vi "Configure Command.vi"(8 "error in (no error)":errorcluster, 10 "settings":T2 {"Linked Channels"."Channel Ref in" format="%.0x"}, 11 "command refnum in":T1=18446744073709551615 format="%.0x") -> (0 "error out":errorcluster, 3 "command refnum out":T1=18446744073709551615 format="%.0x")   [LabVIEW 2020, in "Instrument Addon Scripting API.lvlib"]
doc: "Configures a specified command. \n\nIf you want to use Linked Channels with the Command Format string, ensure the Channel Refnums used in the Linked Channels parameter already exist before calling this SubVI. \n\nAn error will occur in the following situations:\n- The Command Format string contains duplicate Variable Names. \n- The number of variables in the Command Format string differs from the number of Linked Channels. \n- The Variable Names in the Command Format string differs from the names used in the Linked Channels parameter."
uses:
  Instrument Addon Scripting API.lvlib
  TypeDefs/Command Settings.ctl
  <vilib>/NI VeriStand/Custom Device API/Custom Device Item Ref.ctl
  TypeDefs/Padding.ctl
  Addon/Addon Shared/Types/FG Control.ctl
  Addon/Addon Shared/Types/Command Parameters.ctl
  Addon/Addon Shared/Types/Linked Channel Cluster.ctl
  Addon/Addon Shared/SubVIs/Constants.vi
  <vilib>/NI VeriStand/Custom Device API/NI VeriStand - Get Item Property.vi
  <vilib>/NI VeriStand/Custom Device API/Get Item Property (String).vi
  <vilib>/NI VeriStand/Custom Device API/Get Item Property (String Array).vi
  <vilib>/NI VeriStand/Custom Device API/Get Item Property (Boolean).vi
  <vilib>/NI VeriStand/Custom Device API/Get Item Property (U32).vi
  <vilib>/NI VeriStand/Custom Device API/NI VeriStand - Set Item Property.vi
  <vilib>/NI VeriStand/Custom Device API/Set Item Property (String).vi
  <vilib>/NI VeriStand/Custom Device API/Set Item Property (String Array).vi
  <vilib>/NI VeriStand/Custom Device API/Set Item Property (Boolean).vi
  <vilib>/NI VeriStand/Custom Device API/Set Item Property (U32).vi
  Addon/Addon Shared/Instrument Addon Shared.lvlib
  <vilib>/NI VeriStand/Custom Device API/Custom Device API.lvlib
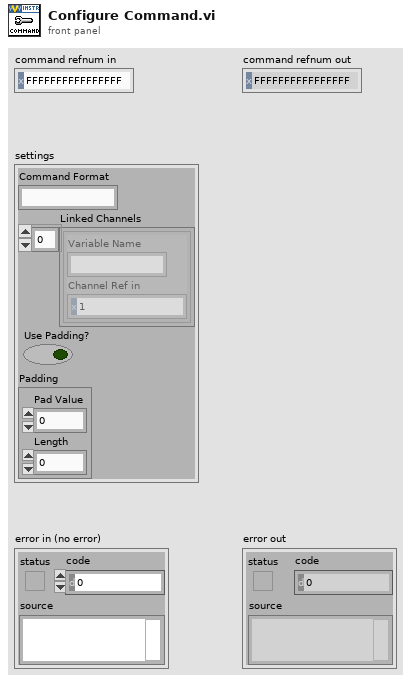
[diagram p1: front panel]
types:
  T1 = typedef "Custom Device API.lvlib/Custom Device Item Ref.ctl" = u64
  T2 = typedef "Instrument Addon Scripting API.lvlib/Command Settings.ctl" = cluster{"Command Format":string, "Linked Channels":cluster{"Variable Name":string, "Channel Ref in":T1}[], "Use Padding?":bool, "Padding":T3}
  T3 = typedef "Instrument Addon Scripting API.lvlib/Padding.ctl" = cluster{"Pad Value":u8, "Length":u32}
  T4 = typedef "Instrument Addon Shared.lvlib/Command Parameters.ctl" = cluster{"Command":string, "Linked Channels":T5[], "Pad":bool, "Length":u32, "Pad Value":u8}
  T5 = typedef "Instrument Addon Shared.lvlib/Linked Channel Cluster.ctl" = cluster{"Variable Name":string, "GUID":string}
  T6 = typedef "Instrument Addon Shared.lvlib/FG Control.ctl" = enum16{"Get", "Set"}
  T7 = cluster{"Variable Name":string, "Channel Ref in":T1}[]
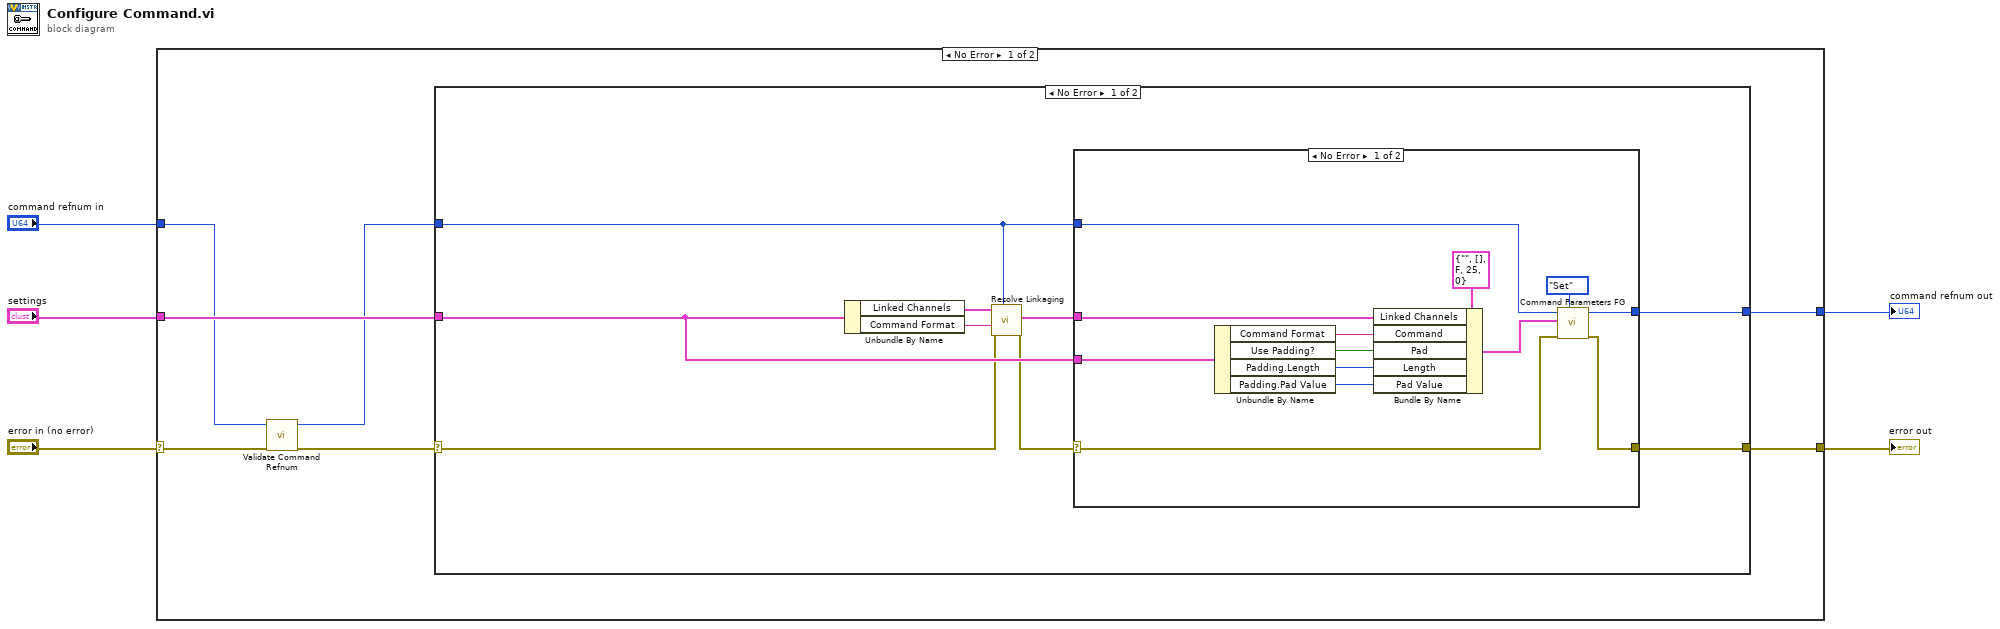
[diagram p0: block diagram]
diagram:
  n1 = case shown="No Error" "error in (no error)" {
    selector: "error in (no error)" -> [w8 w40]
    tunnel: "command refnum in" -> [w9 w39]
    tunnel: "settings" -> [w12 _]
    tunnel: [w11 w40] -> w4
    tunnel: [w10 w39] -> w2
    frame No Error {
      n2 = call "Validate Command Refnum.vi"("error in (no error)"=w8, "command refnum in"=w9) -> ("error out"=w7:errorcluster, "command refnum out"=w6:T1)  [unwired: 8 in]
      n3 = case shown="No Error" w7 {
        selector: w7 -> [w19 w38]
        tunnel: w12 -> [w21 _]
        tunnel: [w20 w38] -> w11
        tunnel: w6 -> [w13 w37]
        tunnel: [w14 w37] -> w10
        frame No Error {
          n4 = Unbundle By Name(w21) -> ("Linked Channels"=w17:T7, "Command Format"=w18:string)
          n5 = call "Resolve Linkaging.vi"("Command/Response Refnum in"=w13, "error in (no error)"=w19, "Command/Response Format"=w18, "Linked Channels"=w17) -> ("error out"=w16:errorcluster, "Linked Channels out"=w15:T5[])  [unwired: 6 in]
          n6 = case shown="No Error" w16 {
            selector: w16 -> [w29 w36]
            tunnel: w15 -> [w27 _]
            tunnel: [w33 w36] -> w20
            tunnel: w13 -> [w34 w35]
            tunnel: w21 -> [w30 _]
            tunnel: [w22 w35] -> w14
            frame No Error {
              n7 = Unbundle By Name(w30) -> ("Command Format"=w26:string, "Use Padding?"=w25:bool, "Padding.Length"=w24:u32, "Padding.Pad Value"=w23:u8)
              n8 = Bundle By Name(cluster=T4 {"Command"="", "Linked Channels"=[], "Pad"=FALSE, "Length"=25, "Pad Value"=0} ("Command Parameters"), "Linked Channels"=w27, "Command"=w26, "Pad"=w25, "Length"=w24, "Pad Value"=w23) -> (w28:T4)
              n9 = call "Command Parameters FG.vi"("Action"=FG_Control."Set", "error in (no error)"=w29, "Command Parameters"=w28, "Item Ref in"=w34) -> ("error out"=w33:errorcluster, "Item Ref out"=w22:T1)  [unwired: 5 in, 1 out]
            }
            frame Error {
            }
          }
        }
        frame Error {
        }
      }
    }
    frame Error {
    }
  }
  "error out" <- w4
  "command refnum out" <- w2
